vi "RSZVB Channel Trace Export Data With Options.vi"(5 "File Name (Trc1.s1p)":string="Trc1.s1p", 6 "Export Data (0: Complex Values)":i32(ring) items=["Complex Values", "Linear magnitude and phase", "dB-magnitude and phase"], 7 "Export Format (0: Unformatted)":i32(ring) items=["Unformatted", "Formatted"], 8 "error in (no error)":errorcluster {"code" format="%.0x"}, 9 "Channel (Trace) (1)":i32=1, 10 "Select Channel (0: Single)":i32(ring) items=["Single", "All"], 11 "VISA session":refnum<visa-resource-name>) -> (0 "error out":errorcluster {"code" format="%.0x"}, 3 "dup VISA session":refnum<visa-resource-name>)   [LabVIEW 2011]
doc: "This VI stores the trace data of all data traces in the specified channel to a trace file.\n\nNote(s):\n\nTraces are created using the CALCulte<Ch>:PARameter:SDEFine... command.\n\n*.s<n>p Touchstone files (<n> = 1, 2, 3, ...) are intended for a complete set of <n>-port S-parameters. Data export fails if the active channel does not contain the full set of <n>^2 traces. \n\n\nRemote-control command(s):\nMMEMory:STORe:TRACe:CHANnel <ch_number> | ALL,'<file_name>'[,UNFormatted | FORMatted, COMPlex | LINPhase | LOGPhase]"
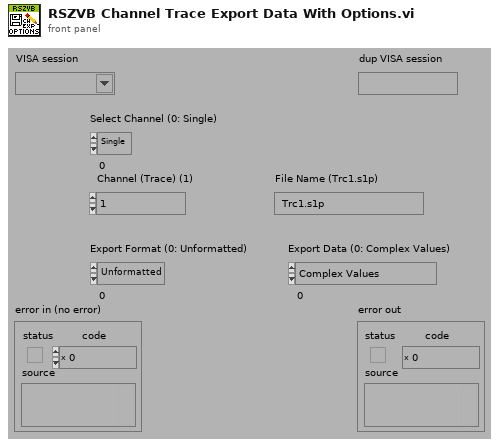
[diagram p1: front panel]
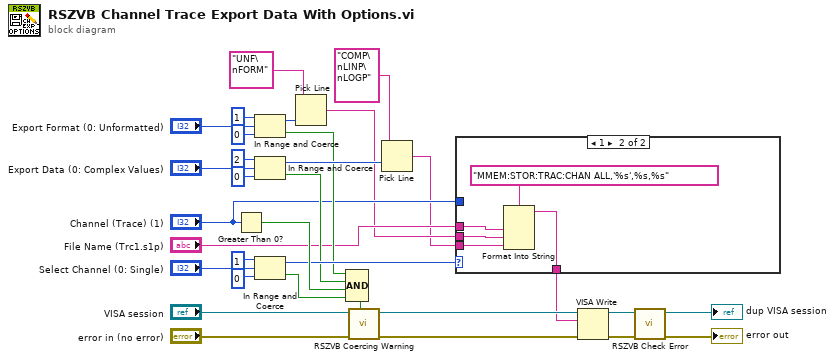
[diagram p0: block diagram]
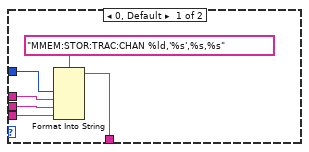
[diagram p2: hidden frame]
diagram:
  n1 = Greater Than 0?(x="Channel (Trace) (1)") -> (x > 0?=w28:bool)
  n2 = In Range and Coerce(upper limit=1, x="Export Format (0: Unformatted)", lower limit=0) -> (coerced(x)=w19:i32, In Range?=w6:bool)
  n3 = In Range and Coerce(upper limit=2, x="Export Data (0: Complex Values)", lower limit=0) -> (coerced(x)=w18:i32, In Range?=w5:bool)
  n4 = In Range and Coerce(upper limit=1, x="Select Channel (0: Single)", lower limit=0) -> (coerced(x)=w8:i32, In Range?=w29:bool)
  n5 = Pick Line(multi-line string="UNF\nFORM", line index=w19) -> (output string=w2:string)  [unwired: 1 in]
  n6 = Compound Arithmetic op=AND(w6, w5, w28, w29) -> (w32:bool)
  n7 = call "RSZVB Coercing Warning.vi"("In Range?"=w32, "error in (no error)"="error in (no error)", "VISA session"="VISA session") -> ("error out"=w12:errorcluster, "dup VISA session"=w17:refnum<visa-resource-name>)  [unwired: 7 in]
  n8 = Pick Line(multi-line string="COMP\nLINP\nLOGP", line index=w18) -> (output string=w1:string)  [unwired: 1 in]
  n9 = case shown="1" w8 {
    tunnel: [w38 w43] -> w7
    tunnel: "Channel (Trace) (1)" -> [w36 _]
    tunnel: "File Name (Trc1.s1p)" -> [w35 w41]
    tunnel: w2 -> [w34 w40]
    tunnel: w1 -> [w33 w39]
    frame 0, Default {
      n10 = Format Into String(format string="MMEM:STOR:TRAC:CHAN %ld,'%s',%s,%s", w36, w35, w34, w33) -> (resulting string=w38:string)  [unwired: 2 in, 1 out]
    }
    frame 1 {
      n11 = Format Into String(format string="MMEM:STOR:TRAC:CHAN ALL,'%s',%s,%s", w41, w40, w39) -> (resulting string=w43:string)  [unwired: 2 in, 1 out]
    }
  }
  n12 = VISA Write(VISA resource name=w17, write buffer=w7, error in (no error)=w12) -> (VISA resource name out=w16:refnum<visa-resource-name>, error out=w13:errorcluster)  [unwired: 1 out]
  n13 = call "RSZVB Check Error.vi"("error in (no error)"=w13, "VISA session"=w16) -> ("error out"=→"error out":errorcluster, "dup VISA session"=→"dup VISA session":refnum<visa-resource-name>)  [unwired: 8 in]
